vi "Pump Status.vi"(8 "error in (no error)":errorcluster, 11 "VICI Settings":T1 {"Pump Number" min=1.0 max=20.0 step=1.0}) -> (0 "error out":errorcluster, 1 "Connection Error":bool, 2 "Pump On?":enum16{"Off", "On", "Not Initialized"}(ring), 3 "VICI Settings":T1 {"Pump Number" min=1.0 max=20.0 step=1.0})   [LabVIEW 2018, in "VICI M50.lvlib"]
uses:
  VICI M50.lvlib
  Settings Cluster.ctl
  <vilib>/Instr/_visa.llb/VISA Flush IO Buffer Mask.ctl
  <vilib>/Instr/_visa.llb/VISA Configure Serial Port (Instr).vi
panel:
  out "result string":string
  out "read buffer":string
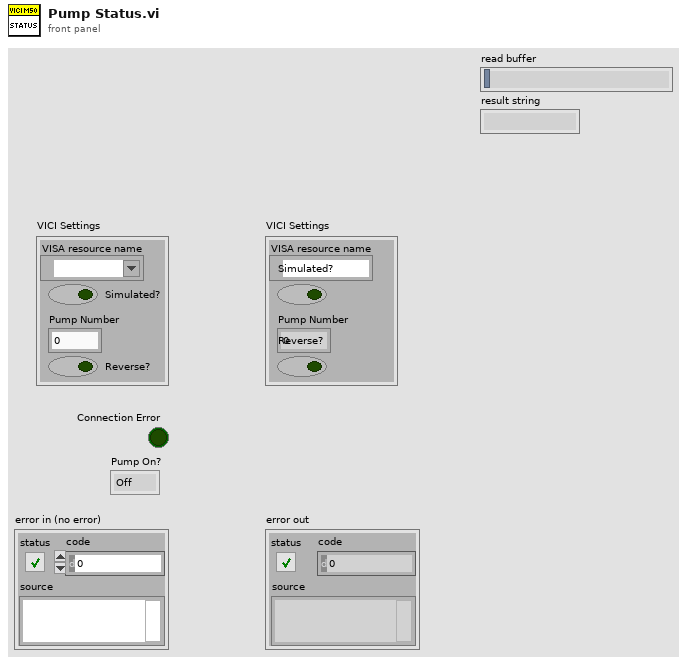
[diagram p1: front panel]
types:
  T1 = typedef "VICI M50.lvlib/Settings Cluster.ctl" = cluster{"VISA resource name":refnum<visa-resource-name>, "Simulated?":bool, "Pump Number":dbl, "Reverse?":bool}
  T2 = typedef "VISA Flush IO Buffer Mask.ctl" = u16
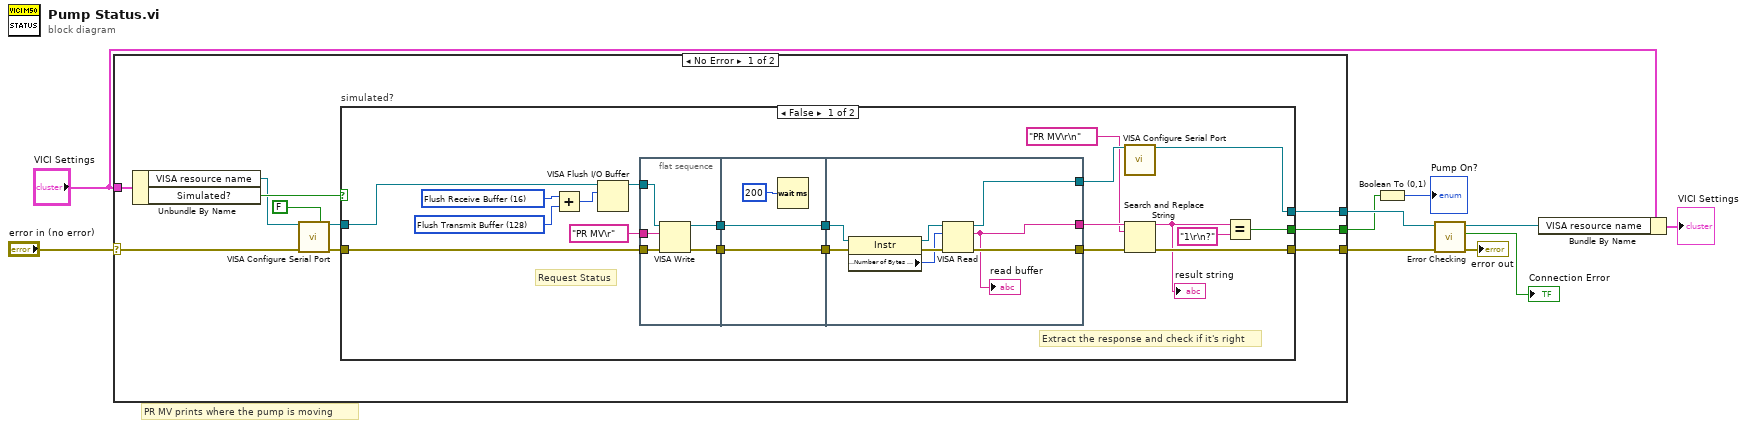
[diagram p0: block diagram]
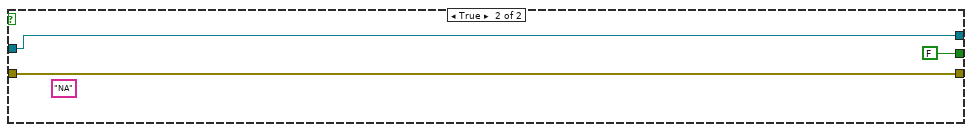
[diagram p2: hidden frame]
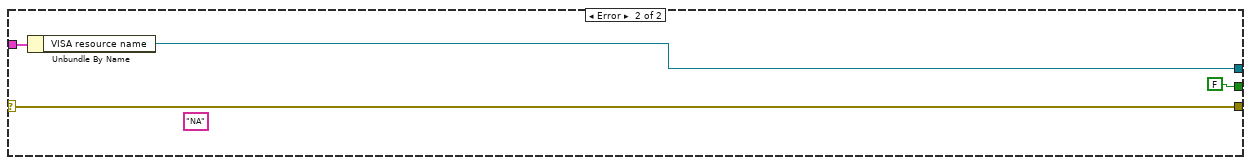
[diagram p3: hidden frame]
diagram:
  # "PR MV prints where the pump is moving"
  n1 = case shown="No Error" "error in (no error)" {
    selector: "error in (no error)" -> [w13 w63]
    tunnel: [w20 w63] -> w8
    tunnel: "VICI Settings" -> [w19 w62]
    tunnel: [w18 w61] -> w5
    tunnel: [w11 FALSE] -> w2
    frame No Error {
      n2 = Unbundle By Name(w19) -> ("VISA resource name"=w16:refnum<visa-resource-name>, "Simulated?"=w17:bool)
      n3 = call-poly "VISA Configure Serial Port"("VISA resource name"=w16, "Enable Termination\nChar (T)"=FALSE ("Enable Termination\nChar (T)"), "error in (no error)"=w13) -> ("VISA resource name out"=w15:refnum<visa-resource-name>, "error out"=w12:errorcluster)  [unwired: 11 in]
      n4 = case "simulated?" shown="False" w17 {
        tunnel: [w24 w59] -> w20
        tunnel: [w28 w57] -> w18
        tunnel: w12 -> [w40 w59]
        tunnel: w15 -> [w34 w57]
        tunnel: [w21 FALSE] -> w11
        frame False {
          w30 = T2 128 items=["Flush Receive Buffer"=16, "Write Transmit Buffer to Device"=32, "Flush Receive Buffer (No I/O)"=64, "Flush Transmit Buffer"=128] ("Mask")
          w31 = T2 16 items=["Flush Receive Buffer"=16, "Write Transmit Buffer to Device"=32, "Flush Receive Buffer (No I/O)"=64, "Flush Transmit Buffer"=128] ("Mask")
          # "Extract the response and check if it's right"
          # "Request Status"
          n5 = Add(x=w31, y=w30) -> (x+y=w32:T2)
          n6 = VISA Flush I/O Buffer(VISA resource name=w34, mask (16)=w32) -> (VISA resource name out=w33:refnum<visa-resource-name>)  [unwired: 1 in, 1 out]
          n7 = flat-sequence {
            tunnel: [w43] -> w39
            tunnel: [w44] -> w38
            tunnel: w40 -> [w41]
            tunnel: "PR MV\r" ("string") -> [w45]
            tunnel: w33 -> [w42]
            tunnel: w39 -> [w46]
            tunnel: w38 -> [w48]
            tunnel: [w48] -> w37
            tunnel: [w46] -> w36
            tunnel: w37 -> [w55]
            tunnel: w36 -> [w54]
            tunnel: [w50] -> w27
            tunnel: [w56] -> w25
            tunnel: [w49] -> w29
            frame #0 {
              n8 = VISA Write(VISA resource name=w42, write buffer=w45, error in (no error)=w41) -> (VISA resource name out=w43:refnum<visa-resource-name>, error out=w44:errorcluster)  [unwired: 1 out]
            }
            frame #1 {
              n9 = Wait (ms)(milliseconds to wait=u32 200) -> ()  [unwired: 1 out]
            }
            frame #2 {
              n10 = property class="Instr"(reference=w54, error in=w55) -> (reference out=w53:refnum<visa-resource-name>, error out=w52:errorcluster, "Serial Settings:Number of Bytes at Serial Port"=w51:u32)
              n11 = VISA Read(VISA resource name=w53, byte count=w51, error in (no error)=w52) -> (VISA resource name out=w49:refnum<visa-resource-name>, read buffer=w50:string, error out=w56:errorcluster)  [unwired: 1 out]
              "read buffer" <- w50
            }
          }
          n12 = call-poly "VISA Configure Serial Port"("VISA resource name"=w29) -> ("VISA resource name out"=w28:refnum<visa-resource-name>)  [unwired: 13 in, 1 out]
          n13 = Search and Replace String(input string=w27, search string="PR MV\r\n", error in=w25) -> (result string=w23:string, error out=w24:errorcluster)  [unwired: 5 in, 2 out]
          "result string" <- w23
          n14 = Equal?(x=w23, y="1\r\n?") -> (x = y?=w21:bool)
        }
        frame True {
          (unwired) "NA" ("read buffer")
        }
      }
    }
    frame Error {
      (unwired) "NA" ("read buffer")
      n15 = Unbundle By Name(w62) -> ("VISA resource name"=w61:refnum<visa-resource-name>)
    }
  }
  n16 = Boolean To (0,1)(Boolean=w2) -> (0, 1=→"Pump On?":i16)
  n17 = call "Error Checking.vi"("error in (no error)"=w8, "VISA resource name"=w5) -> ("error out"=→"error out":errorcluster, "Connection Error"=→"Connection Error":bool, "VISA resource name"=w4:refnum<visa-resource-name>)  [unwired: 7 in]
  n18 = Bundle By Name(cluster="VICI Settings", "VISA resource name"=w4) -> (→"VICI Settings":T1)
